vi "Sound recording example.vi"() -> ()   [LabVIEW 2022 SP3]
uses:
  <vilib>/Analysis/2dsp.llb/Power Spectrum (DBL).vi
  <vilib>/Analysis/NI_AALPro.lvlib
panel:
  out "Waveform Graph 2":dbl[][](graph)
  out "Waveform Graph":dbl[](graph)
  in  "Resolution (bits)":i32=16
  in  "#Channels":i32=2
  in  "Device":u32
  in  "Sample rate (Hz)":dbl=22050.0
  in  "Duration (s)":dbl=1.0
  out "Data":dynamicdata(graph)
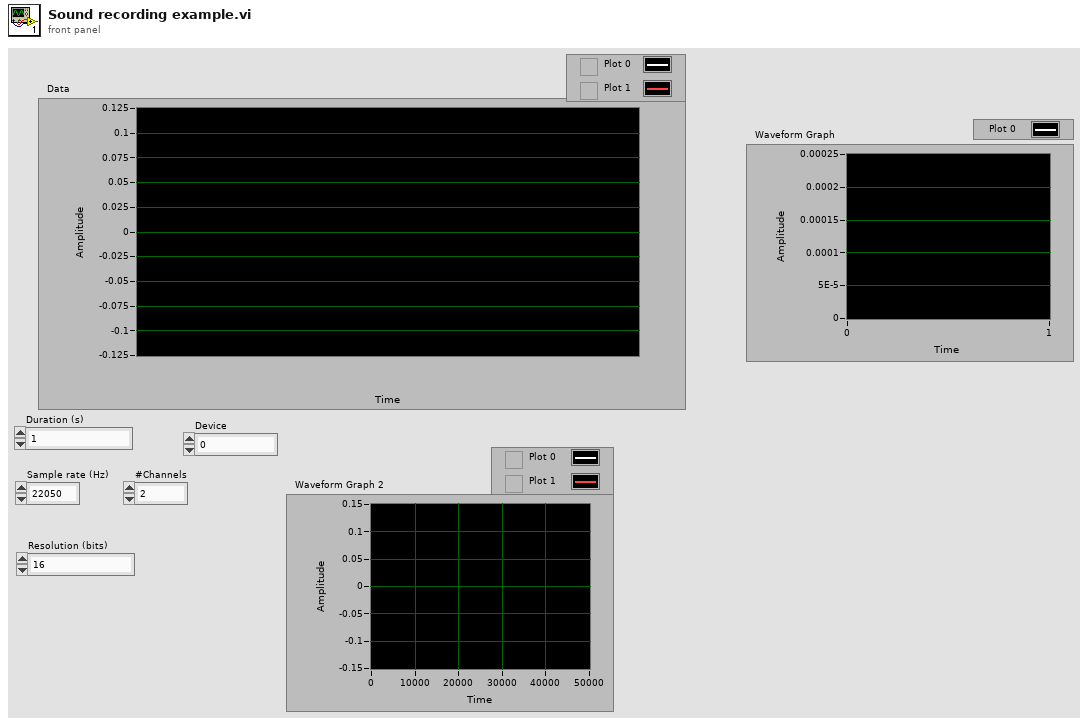
[diagram p1: front panel]
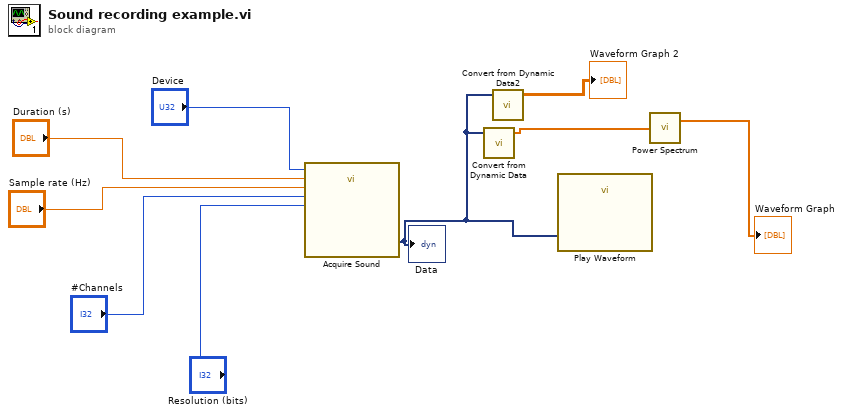
[diagram p0: block diagram]
diagram:
  n1 = call "Acquire Sound"("Device"="Device", "Duration (s)"="Duration (s)", "Sample rate (Hz)"="Sample rate (Hz)", "#Channels"="#Channels", "Resolution (bits)"="Resolution (bits)") -> ("Data"=w2:dynamicdata)  [unwired: 13 in, 1 out]
  "Data" <- w2
  n2 = call "Convert from Dynamic Data"("Dynamic Data Type"=w2) -> ("Array"=w3:dbl[])  [unwired: 3 in]
  n3 = call "Convert from Dynamic Data2"("Dynamic Data Type"=w2) -> ("Array"=→"Waveform Graph 2":dbl[][])  [unwired: 3 in]
  n4 = call "Play Waveform"("Data"=w2) -> ()  [unwired: 18 in, 1 out]
  n5 = call-poly <vilib>:"Power Spectrum.vi"("X"=w3) -> ("Power Spectrum"=→"Waveform Graph":dbl[])  [unwired: 1 out]
